vi "set_x_and_y_move_speeds_Z-tilt.vi"(4 "Switch X and Y (t)":bool=TRUE, 6 "Motor2-xRays (angle)":dbl, 7 "Use standard V_max (f)":bool, 8 "error in (no error)":errorcluster, 9 "rotate by (degrees)":dbl, 10 "V_max total":dbl=15000.0, 11 "VISA resource name":refnum<visa-resource-name>) -> (0 "error out":errorcluster={"status"=FALSE, "code"=1073676294, "source"="VISA Read in write_read.vi"}, 1 "V_max Motor 2":i32, 2 "V_max Motor 1":i32, 3 "VISA ressource out":refnum<visa-resource-name>)   [LabVIEW 2013]
uses:
  MCode_LV_86/Set Parameter.ctl
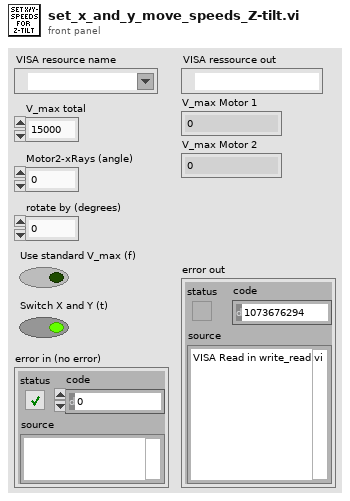
[diagram p1: front panel]
types:
  T1 = typedef "Set Parameter.ctl" = enum16{"Acceleration (A)", "Baud Rate (BD)", "Counter 1 (C1)", "Counter 2 (C2)", "Control C Software Reset (CE)", "Check Sum Enable (CK)", "Clock Mode (CM)", "Clock Mode Ratio (CR)", "Clock Mode Out Step Width (CW)", "Deceleration (D)", "Digital Filtering, Input 1 (D1)", "Digital Filtering, Input 2 (D2)", "Digital Filtering, Input 3 (D3)", "Digital Filtering, Input 4 (D4)", "Digital Filtering, Input 5 (D5)", "Digital Filtering, Input 9 (D9)", "Digital Filtering, Input 10 (D10)", "Digital Filtering, Input 11 (D11)", "Digital Filtering, Input 12 (D12)", "Deadband (DB)", "Decrement Variable (DC)", "Enable/Disable Drive (DE)", "Device Name (DN)", "End Program Execution (E)", "Encoder Function Enable (EE)", "Encoder Lines (EL)", "Echo Mode (EM)", "Error Value (ER)", "Escape (ES)", "Execute Program at Address (EX)", "Firmware Version (VR)", "Hold (H)", "Hold Current (HC)", "Hold Current Delay Time (HI)", "Home to Encoder Index (HM)", "Home to Home Switch (HT)", "Increment Variable (IC)", "Initialize Parameters to NVM (IP)", "Input into Variable (IV)", "Jog Enable (JE)", "Limit Stop Mode (LM)", "Move Absolute (MA)", "Move Relative (MR)", "MicroStepping Select (MS)", "Motor Settling Delay Time (MT)", "Moving [Flag] (MV)", "Output 1 (O1)", "Output 2 (O2)", "Output 3 (O3)", "Output 4 (O4)", "Output 9 (O9)", "Output 10 (O10)", "Output 11 (O11)", "Output 12 (O12)", "Output High Byte (9-12) (OH)", "Output Low Byte (1-4) (OL)", "Output Total (1-4 and 9-12) (OT)", "Position (P)", "Position Maintenance (PM)", "Party Mode (PY)", "Register 1 (R1)", "Register 2 (R2)", "Register 3 (R3)", "Register 4 (R4)", "Reset Error(\\03)", "Run Current (RC)", "Stall Factor (SF)", "Slew (SL)", "Stall Mode Set (SM)", "Upgrade Firmware (UG)", "Velocity Initial (VI)", "Velocity Maximum (VM)"}
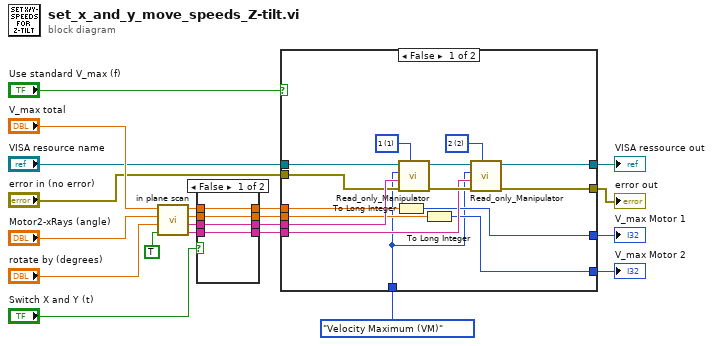
[diagram p0: block diagram]
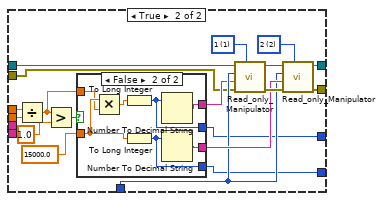
[diagram p3: hidden frame]
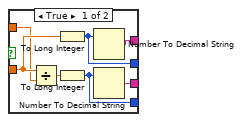
[diagram p4: hidden frame]
diagram:
  n1 = call "in plane scan.vi"("abs(x,y)"=TRUE, "rotate by (degrees)"="rotate by (degrees)", "angle (degrees)"="Motor2-xRays (angle)", "v total"="V_max total") -> ("v_y string"=w6:string, "v_x string"=w8:string, "v_y"=w10:dbl, "v_x"=w12:dbl)  [unwired: 2 in, 2 out]
  n2 = case shown="False" "Switch X and Y (t)" {
    tunnel: w12 -> [w25 w27]
    tunnel: [w25 w26] -> w11
    tunnel: w10 -> [w24 w26]
    tunnel: [w24 w27] -> w9
    tunnel: w8 -> [w23 w29]
    tunnel: [w23 w28] -> w7
    tunnel: w6 -> [w22 w28]
    tunnel: [w22 w29] -> w5
    frame False {
    }
    frame True {
    }
  }
  n3 = case shown="False" "Use standard V_max (f)" {
    tunnel: w7 -> [w42 _]
    tunnel: w5 -> [w41 _]
    tunnel: [w38 w59] -> w20
    tunnel: [w37 w57] -> w19
    tunnel: w11 -> [w36 w56]
    tunnel: [w35 w47] -> w16
    tunnel: w9 -> [w34 w55]
    tunnel: [w33 w46] -> w15
    tunnel: "VISA resource name" -> [w32 w60]
    tunnel: "error in (no error)" -> [w31 w45]
    tunnel: Set_Parameter."Velocity Maximum (VM)" ("Command") -> [w30 w49]
    frame False {
      w40 = u16 1 items=["none", "1", "2", "3", "4", "all"] ("Motor")
      w39 = u16 2 items=["none", "1", "2", "3", "4", "all"] ("Motor")
      n4 = To Long Integer(number=w36) -> (32bit integer=w35:i32)
      n5 = call "Read_only_Manipulator.vi"("Motor"=w40, "error in (no error)"=w31, "Value"=w42, "Command"=w30, "VISA resource name"=w32) -> ("error out"=w44:errorcluster, "VISA ressource out"=w43:refnum<visa-resource-name>)  [unwired: 3 in, 2 out]
      n6 = To Long Integer(number=w34) -> (32bit integer=w33:i32)
      n7 = call "Read_only_Manipulator.vi"("Motor"=w39, "error in (no error)"=w44, "Value"=w41, "Command"=w30, "VISA resource name"=w43) -> ("error out"=w37:errorcluster, "VISA ressource out"=w38:refnum<visa-resource-name>)  [unwired: 3 in, 2 out]
    }
    frame True {
      w62 = u16 1 items=["none", "1", "2", "3", "4", "all"] ("Motor")
      w61 = u16 2 items=["none", "1", "2", "3", "4", "all"] ("Motor")
      n8 = Divide(x=w56, y=w55) -> (x/y=w52:dbl)
      n9 = Greater?(x=w52, y=1.0) -> (0:w53:bool)
      n10 = case shown="False" w53 {
        tunnel: w52 -> [w66 w74]
        tunnel: 15000.0 -> [w67 w75]
        tunnel: [w70 w77] -> w48
        tunnel: [w69 w76] -> w50
        tunnel: [w65 w72] -> w47
        tunnel: [w64 w71] -> w46
        frame True {
          n11 = Divide(x=w67, y=w66) -> (x/y=w68:dbl)
          n12 = To Long Integer(number=w67) -> (32bit integer=w65:i32)
          n13 = To Long Integer(number=w68) -> (32bit integer=w64:i32)
          n14 = Number To Decimal String(number=w65) -> (decimal integer string=w70:string)  [unwired: 1 in]
          n15 = Number To Decimal String(number=w64) -> (decimal integer string=w69:string)  [unwired: 1 in]
        }
        frame False {
          n16 = Multiply(x=w75, y=w74) -> (x*y=w73:dbl)
          n17 = To Long Integer(number=w73) -> (32bit integer=w72:i32)
          n18 = To Long Integer(number=w75) -> (32bit integer=w71:i32)
          n19 = Number To Decimal String(number=w72) -> (decimal integer string=w77:string)  [unwired: 1 in]
          n20 = Number To Decimal String(number=w71) -> (decimal integer string=w76:string)  [unwired: 1 in]
        }
      }
      n21 = call "Read_only_Manipulator.vi"("Motor"=w62, "error in (no error)"=w45, "Value"=w48, "Command"=w49, "VISA resource name"=w60) -> ("error out"=w58:errorcluster, "VISA ressource out"=w63:refnum<visa-resource-name>)  [unwired: 3 in, 2 out]
      n22 = call "Read_only_Manipulator.vi"("Motor"=w61, "error in (no error)"=w58, "Value"=w50, "Command"=w49, "VISA resource name"=w63) -> ("error out"=w57:errorcluster, "VISA ressource out"=w59:refnum<visa-resource-name>)  [unwired: 3 in, 2 out]
    }
  }
  "VISA ressource out" <- w20
  "error out" <- w19
  "V_max Motor 1" <- w16
  "V_max Motor 2" <- w15
